vi "Actor.vi"(4 "Async Elements":refnum<class "Async Elements.lvclass">, 11 "TEMPLATE Actor in":refnum<class "TEMPLATE Actor.lvclass">) -> (0 "Error out":errorcluster, 3 "TEMPLATE Actor out":refnum<class "TEMPLATE Actor.lvclass">)   [LabVIEW 2025, in "_Template.lvlib" / "Templates.lvlib" / "TEMPLATE jettl Actor.lvlib" / "TEMPLATE Actor.lvlib" / "TEMPLATE Actor.lvclass"]
uses:
  TEMPLATE Actor.lvclass
  jettl/jettl/Async Elements/Async Elements.lvclass
  TEMPLATE Refs/Refs.ctl
  TEMPLATE Actor.lvclass/TEMPLATE Actor.ctl
  TEMPLATE Refs/TEMPLATE Refs.lvlib
  jettl/jettl/jettl.lvlib
  jettl/jettl/Event Transport/Event Transport.lvlib
types:
  T1 = typedef "_Template.lvlib/Templates.lvlib/TEMPLATE jettl Actor.lvlib/TEMPLATE Actor.lvlib/TEMPLATE Refs.lvlib/Refs.ctl" = cluster{"placeholder":refnum<vi>}
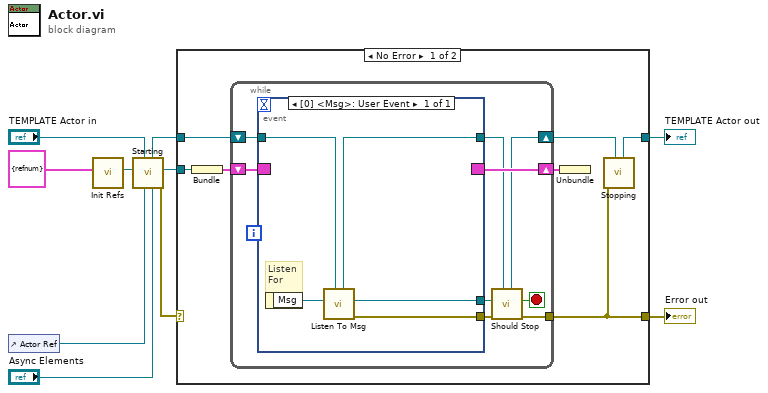
[diagram p0: block diagram]
diagram:
  n1 = control-ref of="Actor Ref"() -> (w3:refnum<vi>)
  n2 = call "Init Refs.vi"("Refs"=T1 {"placeholder"=refnum} ("Control Refs")) -> ("Refs"=w4:refnum<class "Refs.lvclass">)  [unwired: 10 in]
  n3 = call "Starting.vi"("Async Elements"="Async Elements", "VI Ref"=w3, "Actor in"="TEMPLATE Actor in", "Refs"=w4) -> ("Error out"=w5:errorcluster, "Msg Ref"=w2:refnum<event-registration>, "Actor out"=w6:refnum<class "TEMPLATE Actor.lvclass">)  [unwired: 5 in]
  n4 = case shown="No Error" w5 {
    selector: w5 -> [_ w32]
    tunnel: [w15 w33] -> w9
    tunnel: w6 -> [w12 w33]
    tunnel: [w17 w32] -> w10
    tunnel: w2 -> [w11 _]
    frame No Error {
      n5 = Bundle("Msg Ref"=w11) -> (w14:cluster{"Msg Ref":refnum<event-registration>})  [unwired: 1 in]
      n6 = while {
        shift-right: [w19] -> w16
        shift-left: w12 -> [w25]
        tunnel: [w23] -> w17
        shift-right: [w20] -> w13
        shift-left: w14 -> [w26]
        stop <- w22 stop-if-true
        n7 = event shown="[0] <Msg>: User Event" {
          selector: w26 -> [_]
          dyn-events: [_] -> w20
          timeout: _ -> [_]
          tunnel: w25 -> [w31]
          tunnel: [w29] -> w18
          tunnel: [w28] -> w24
          tunnel: [w27] -> w21
          event User Event {
            # "Listen\nFor"
            n8 = event-data() -> ("Msg"=w30:refnum<class "Msg.lvclass">)  [unwired: 1 in]
            n9 = call "Listen To Msg.vi"("Actor in"=w31, "Msg"=w30) -> ("Error out"=w28:errorcluster, "Msg Output"=w27:refnum<class "Msg Output.lvclass">, "Actor out"=w29:refnum<class "TEMPLATE Actor.lvclass">)  [unwired: 7 in]
          }
        }
        n10 = call "Should Stop.vi"("Actor in"=w18, "Error in"=w24, "Msg Output"=w21) -> ("Error out"=w23:errorcluster, "Stop"=w22:bool, "Actor out"=w19:refnum<class "TEMPLATE Actor.lvclass">)  [unwired: 6 in]
      }
      n11 = Unbundle(w13) -> ()  [unwired: 1 out]
      n12 = call "Stopping.vi"("Actor in"=w16, "Error in"=w17) -> ("Actor out"=w15:refnum<class "TEMPLATE Actor.lvclass">)  [unwired: 9 in]
    }
    frame Error {
    }
  }
  "TEMPLATE Actor out" <- w9
  "Error out" <- w10
